vi "Calibration Zero.vi"(8 "error in (no error)":errorcluster, 10 "Platform Slot Number (10)":i16=10 min=-1 max=255, 11 "VISA resource name":refnum<visa-resource-name>) -> (0 "error out":errorcluster, 3 "VISA resource name out":refnum<visa-resource-name>)   [LabVIEW 2018, in "LTB-1.lvlib" / "3150.lvlib"]
doc: "Performs the mechanism of the instrument returning to its home position."
uses:
  3150.lvlib
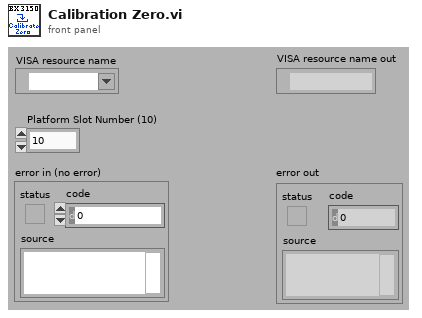
[diagram p1: front panel]
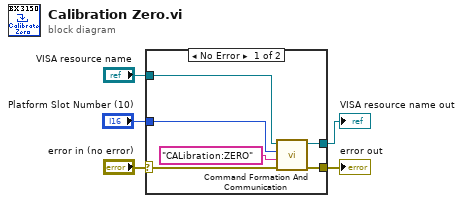
[diagram p0: block diagram]
diagram:
  n1 = case shown="No Error" "error in (no error)" {
    selector: "error in (no error)" -> [w10 w12]
    tunnel: "VISA resource name" -> [w11 w13]
    tunnel: [w9 w13] -> w3
    tunnel: [w8 w12] -> w2
    tunnel: "Platform Slot Number (10)" -> [w6 _]
    frame No Error {
      n2 = call "Command Formation And Communication.vi"("error in (no error)"=w10, "Command"="CALibration:ZERO", "Platform Slot Number"=w6, "VISA resource name"=w11) -> ("error out"=w8:errorcluster, "VISA resource name out"=w9:refnum<visa-resource-name>)  [unwired: 6 out]
    }
    frame Error {
    }
  }
  "VISA resource name out" <- w3
  "error out" <- w2
